vi "Handle Error.vi"(8 "error in (no error)":errorcluster, 11 "Test Actor in":refnum<class "Test Actor.lvclass">) -> (0 "error out":errorcluster, 2 "stop actor?":bool=TRUE, 3 "Test Actor out":refnum<class "Test Actor.lvclass">)   [LabVIEW 2020, in "Test.lvlib" / "Test Actor.lvclass"]
doc: "(<B>Filename</B>: Actor Framework.lvlib:Actor.lvclass:Handle Error.vi)\n\nDefines how the actor handles an error that occurred while processing a message. By default, this method does nothing except stop the actor."
uses:
  Test Actor.lvclass
  <vilib>/event_ctls.llb/usereventprio.ctl
  Test Actor.lvclass/Test Actor.ctl
  PPL/HDH.Actor Framework.Core.Sequencer.lvlibp/Sequencer/Sequencer.lvclass
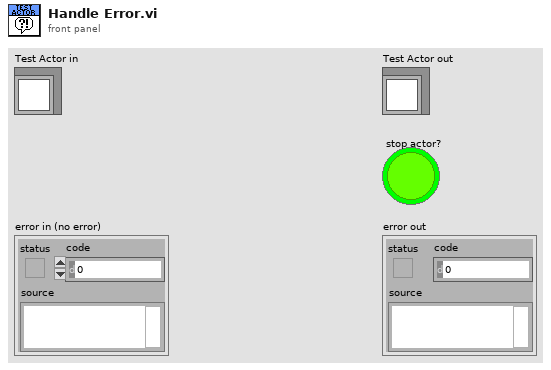
[diagram p1: front panel]
types:
  T1 = typedef "usereventprio.ctl" = enum32{"high priority", "normal priority"}
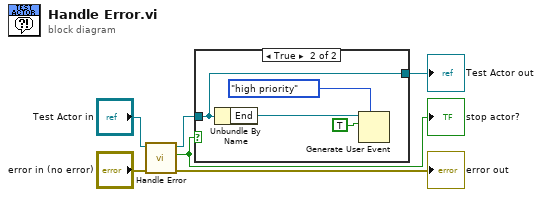
[diagram p0: block diagram]
diagram:
  n1 = call-parent "Handle Error.vi"("error in (no error)"="error in (no error)", "Actor in"="Test Actor in") -> ("error out"=→"error out":errorcluster, "stop actor?"=w3:bool, "Actor out"=w1:refnum<class "Test Actor.lvclass">)  [unwired: 7 in]
  "stop actor?" <- w3
  n2 = case shown="True" w3 {
    tunnel: [w7 w10] -> w2
    tunnel: w1 -> [w7 w10]
    frame False {
    }
    frame True {
      n3 = Unbundle By Name(w10) -> ("End"=w11:refnum<user-event>)
      n4 = Generate User Event(priority (normal)=usereventprio."high priority", user event=w11, event data cluster=TRUE ("event data")) -> ()  [unwired: 1 in, 2 out]
    }
  }
  "Test Actor out" <- w2
